vi "ThrowError.vi"(10 "Error Message":string) -> (2 "error out":errorcluster)   [LabVIEW 2019, in "AssertionTest.lvlib"]
uses:
  AssertionTest.lvlib
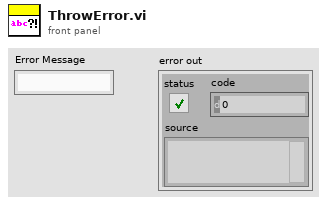
[diagram p1: front panel]
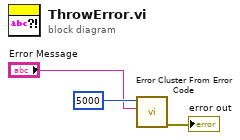
[diagram p0: block diagram]
diagram:
  n1 = call <vilib>:"Error Cluster From Error Code.vi"("error message (\"\")"="Error Message", "error code (0)"=5000) -> ("error out"=→"error out":errorcluster)  [unwired: 7 in]
